vi "Edit Line.vi"(8 "error in":errorcluster, 10 "Line Name":string, 11 "References":T1) -> (0 "error out":errorcluster, 2 "change?":bool)   [LabVIEW 2015, in "TDMS datalogger editor node.lvclass"]
uses:
  TDMS datalogger editor node.lvclass
  <vilib>/NI/DCAF/Tag Editor Core/Table API/Table Manager/object ref.ctl
  <vilib>/NI/DCAF/Tag Editor Core/Configuration Editor/Classes/Engine Parent/Engine Parent Editor Node.lvclass
  <vilib>/NI/DCAF/Tag Editor Core/Configuration Editor/Classes/Module editor node/module editor node.lvclass
  module/configuration/TDMS datalogger configuration.lvclass
  <vilib>/NI/Configuration Framework/serializable configuration/NISE_CEF_serializable configuration.lvclass/NISE_CEF_serializable configuration.ctl
  <vilib>/Utility/LVClass/Get LV Class Name.vi
  <vilib>/NI/Configuration Framework/error generator/NISE_error generator.vi
  <vilib>/NI/Configuration Framework/serializable configuration/NISE_CEF_serializable configuration.lvclass
  <vilib>/NI/DCAF/Tag Editor Core/Table API/Table Manager/Table Manager.lvclass
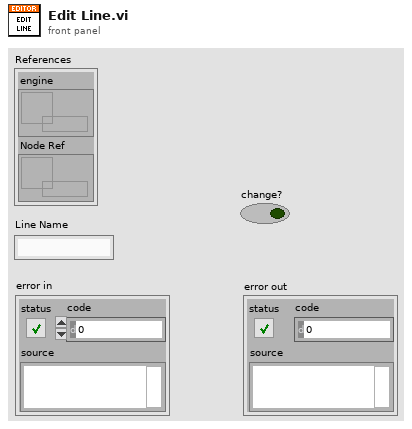
[diagram p1: front panel]
types:
  T1 = typedef "Table Manager.lvlib/Table Manager.lvclass/object ref.ctl" = cluster{"engine":refnum<data-value>, "Node Ref":refnum<data-value>}
  T2 = cluster{"channel":refnum<class "TBM channel.lvclass">}[]
  T3 = cluster{"channel":refnum<class "TBM channel.lvclass">}
  T4 = cluster{"Line":cluster{"channel":refnum<class "TBM channel.lvclass">}, "Maps":cluster{"tag name":string, "channel":refnum<class "TBM channel.lvclass">}[]}
  T5 = cluster{"tag name":string, "channel":refnum<class "TBM channel.lvclass">}[]
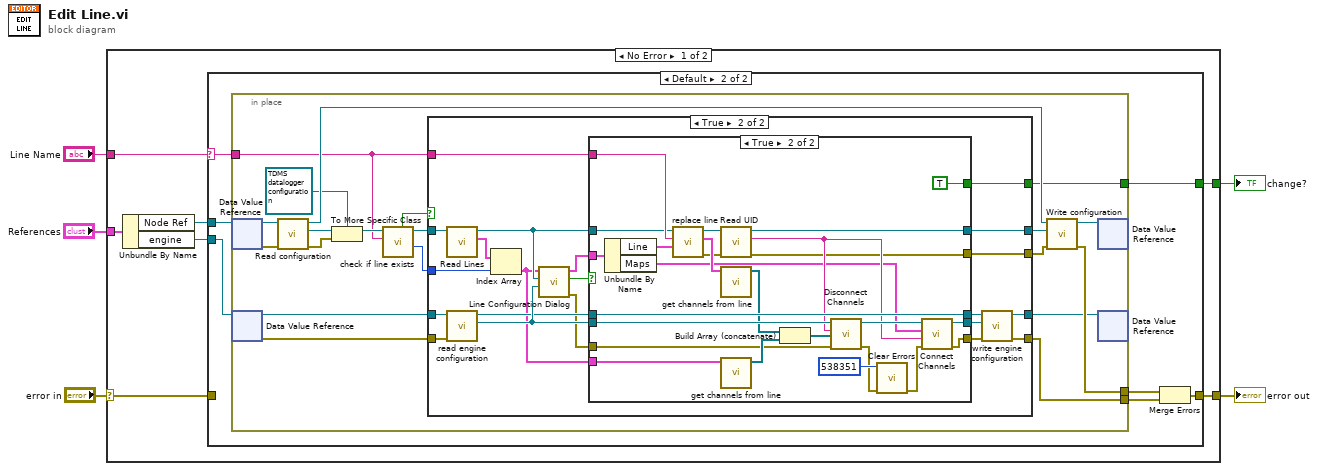
[diagram p0: block diagram]
diagram:
  n1 = case shown="No Error" "error in" {
    selector: "error in" -> [w6 w94]
    tunnel: "References" -> [w10 _]
    tunnel: "Line Name" -> [w7 _]
    tunnel: [w9 w94] -> w2
    tunnel: [w8 _] -> w1
    frame No Error {
      n2 = Unbundle By Name(w10) -> ("Node Ref"=w12:refnum<data-value>, "engine"=w11:refnum<data-value>)
      n3 = case shown="Default" w7 {
        selector: w7 -> [_ w14]
        tunnel: w12 -> [_ w20]
        tunnel: w11 -> [_ w19]
        tunnel: [w13 w16] -> w9
        tunnel: [_ w15] -> w8
        tunnel: w6 -> [w13 _]
        frame " " {
        }
        frame Default {
          n4 = in-place {
            in-place-border: [w29] -> w18
            in-place-border: [w23] -> w17
            in-place-border: [w28] -> w15
            in-place-border: w14 -> [w33]
            n5 = in-place-dvr #1(w20) -> (w39:refnum<class "module editor node.lvclass">, w34:errorcluster)
            n6 = in-place-dvr #2(w19) -> (w26:refnum<class "Engine Parent Editor Node.lvclass">, w25:errorcluster)
            n7 = call-dynamic "Read configuration.vi"("error in"=w34, "NISE_CEF_serializable node in"=w39) -> ("error out"=w36:errorcluster, "configuration"=w37:refnum<class "NISE_CEF_serializable configuration.lvclass">, "NISE_CEF_serializable node out"=w38:refnum<class "module editor node.lvclass">)  [unwired: 7 in]
            n8 = To More Specific Class(target class=refnum<class "TDMS datalogger configuration.lvclass"> refnum ("TDMS datalogger configuration"), reference=w37, error in=w36) -> (specific class reference=w35:refnum<class "TDMS datalogger configuration.lvclass">)  [unwired: 1 out]
            n9 = call "check if line exists.vi"("Name to Locate"=w33, "TDMS datalogger configuration"=w35) -> ("Index"=w30:i32, "TDMS datalogger configuration"=w31:refnum<class "TDMS datalogger configuration.lvclass">, "Found?"=w27:bool)  [unwired: 5 in, 2 out]
            n10 = case shown="True" w27 {
              tunnel: w31 -> [w43 w63]
              tunnel: w33 -> [_ w64]
              tunnel: [w43 w58] -> w32
              tunnel: w30 -> [_ w60]
              tunnel: [_ w56] -> w28
              tunnel: w26 -> [w42 w55]
              tunnel: w25 -> [w41 w54]
              tunnel: [w42 w52] -> w24
              tunnel: [w41 w51] -> w23
              tunnel: [_ w44] -> w22
              frame False {
              }
              frame True {
                n11 = call-dynamic "Read Lines.vi"("TDMS datalogger configuration in"=w63) -> ("Lines"=w61:T2, "TDMS datalogger configuration out"=w62:refnum<class "TDMS datalogger configuration.lvclass">)  [unwired: 8 in, 1 out]
                n12 = call <vilib>:"read engine configuration.vi"("error in"=w54, "Engine Parent Editor Node in"=w55) -> ("engine configuration"=w53:refnum<class "engine configuration.lvclass">, "Engine Parent Editor Node out"=w49:refnum<class "Engine Parent Editor Node.lvclass">)  [unwired: 7 in, 1 out]
                n13 = Index Array(array=w61, index=w60) -> (element=w45:T3)
                n14 = call "Line Configuration Dialog.vi"("engine configuration in"=w53, "TDMS datalogger configuration"=w62, "Line"=w45) -> ("error out"=w46:errorcluster, "changed"=w57:bool, "Mappings out"=w59:T4)  [unwired: 5 in, 1 out]
                n15 = case shown="True" w57 {
                  tunnel: w64 -> [_ w93]
                  tunnel: w53 -> [w67 w92]
                  tunnel: w62 -> [w68 w89]
                  tunnel: w59 -> [_ w88]
                  tunnel: [w68 w86] -> w58
                  tunnel: [_ TRUE ("change?")] -> w56
                  tunnel: [w67 w83] -> w48
                  tunnel: [w66 w82] -> w50
                  tunnel: w49 -> [w66 w82]
                  tunnel: [w65 w80] -> w47
                  tunnel: w46 -> [w65 w75]
                  tunnel: w45 -> [_ w71]
                  tunnel: [_ w69] -> w44
                  frame False {
                  }
                  frame True {
                    n16 = Unbundle By Name(w88) -> ("Line"=w87:T3, "Maps"=w79:T5)
                    n17 = call "replace line.vi"("Line"=w87, "Line Name"=w93, "TDMS datalogger configuration"=w89) -> ("error out"=w70:errorcluster, "Old Line"=w90:T3, "TDMS datalogger configuration out"=w91:refnum<class "TDMS datalogger configuration.lvclass">)  [unwired: 6 in]
                    n18 = call <vilib>:"Read UID.vi"("error in"=w70, "configuration in"=w91) -> ("error out"=w69:errorcluster, "instance id"=w81:string, "configuration out"=w86:refnum<class "TDMS datalogger configuration.lvclass">)  [unwired: 7 in]
                    n19 = call "get channels from line.vi"("Line"=w90) -> ("Channels"=w78:refnum<class "TBM channel.lvclass">[])  [unwired: 10 in]
                    n20 = call "get channels from line.vi"("Line"=w71) -> ("Channels"=w77:refnum<class "TBM channel.lvclass">[])  [unwired: 10 in]
                    n21 = Build Array (concatenate)(w78, w77) -> (w76:refnum<class "TBM channel.lvclass">[])
                    n22 = call "Disconnect Channels.vi"("error in (no error)"=w75, "Deleted Channels"=w76, "instance id"=w81, "Engine Configuration in"=w92) -> ("error out"=w73:errorcluster, "Engine Configuration out"=w85:refnum<class "engine configuration.lvclass">)  [unwired: 6 in]
                    n23 = call <vilib>:"Clear Errors.vi"("error in (no error)"=w73, "specific error code to clear (0: all)"=538351) -> ("error out"=w72:errorcluster)  [unwired: 4 in, 1 out]
                    n24 = call "Connect Channels.vi"("error in (no error)"=w72, "instance id"=w81, "Maps"=w79, "Engine Configuration in"=w85) -> ("error out"=w80:errorcluster, "Engine Configuration out"=w83:refnum<class "engine configuration.lvclass">)  [unwired: 6 in]
                  }
                }
                n25 = call <vilib>:"write engine configuration.vi"("error in"=w47, "engine configuration"=w48, "Engine Parent Editor Node in"=w50) -> ("error out"=w51:errorcluster, "Engine Parent Editor Node out"=w52:refnum<class "Engine Parent Editor Node.lvclass">)  [unwired: 7 in]
              }
            }
            n26 = call-dynamic "Write configuration.vi"("error in"=w22, "configuration"=w32, "NISE_CEF_serializable node in"=w38) -> ("error out"=w29:errorcluster, "NISE_CEF_serializable node out"=w40:refnum<class "module editor node.lvclass">)  [unwired: 7 in]
            n27 = in-place-dvr #1(w40) -> ()  [unwired: 2 out]
            n28 = in-place-dvr #2(w24) -> ()  [unwired: 2 out]
          }
          n29 = Merge Errors(w18, w17) -> (w16:errorcluster)
        }
      }
    }
    frame Error {
    }
  }
  "change?" <- w1
  "error out" <- w2
